vi "Get Scan Engine CD from Target.vi"(8 "error in":errorcluster, 11 "Item Ref in":T1 format="%.0x") -> (0 "error out":errorcluster, 1 "scan engine custom device ref":T1 format="%.0x", 3 "Item Ref out":T1 format="%.0x")   [LabVIEW 2026, in "SEECD System Explorer.lvlib"]
uses:
  SEECD System Explorer.lvlib
  <vilib>/NI VeriStand/Custom Device Tools/Custom Device Utility Library/Custom Device Utility Library.lvlib
  <vilib>/NI VeriStand/Custom Device Offline API/Custom Device Offline API.lvlib
  Scripting/Scan Engine Scripting.lvlib
  C:/Users/Administrator/Desktop/Jatin/All DNC DLLs/NationalInstruments.VeriStand.SystemDefinitionAPI.dll
  Jatin/All DNC DLLs/NationalInstruments.VeriStand.SystemDefinitionAPI.dll
  <vilib>/NI VeriStand/Custom Device API/Custom Device Item Ref.ctl
  <vilib>/NI VeriStand/Custom Device API/Custom Device API.lvlib
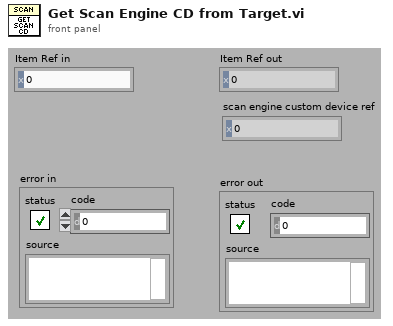
[diagram p1: front panel]
types:
  T1 = typedef "Custom Device API.lvlib/Custom Device Item Ref.ctl" = u64
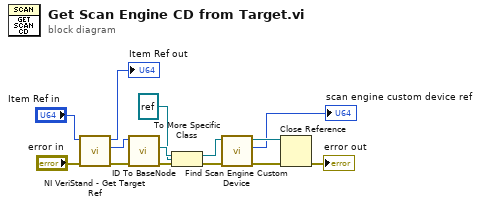
[diagram p0: block diagram]
diagram:
  n1 = call <vilib>:"NI VeriStand - Get Target Ref.vi"("error in"="error in", "Item Ref in"="Item Ref in") -> ("error out"=w6:errorcluster, "Target Ref"=w10:T1, "Item Ref out"=→"Item Ref out":T1)  [unwired: 6 in, 1 out]
  n2 = call <vilib>:"ID To BaseNode.vi"("error in (no error)"=w6, "ID in"=w10) -> ("error out"=w9:errorcluster, "BaseNode"=w8:refnum<k24>)  [unwired: 7 in, 1 out]
  n3 = To More Specific Class(target class=refnum<k39> refnum, reference=w8, error in=w9) -> (specific class reference=w4:refnum<k39>, error out=w5:errorcluster)
  n4 = call "Find Scan Engine Custom Device.vi"("error in"=w5, "NationalInstruments.VeriStand.SystemDefinitionAPI.Target"=w4) -> ("error out"=w2:errorcluster, "scan engine custom device ref"=→"scan engine custom device ref":T1, "NationalInstruments.VeriStand.SystemDefinitionAPI.Target"=w3:refnum<k39>)  [unwired: 6 in, 1 out]
  n5 = Close Reference(reference=w3, error in (no error)=w2) -> (error out=→"error out":errorcluster)
